vi "Update All.vi"(0 "reference in":refnum<class "AI.lvclass">, 5 "error in (no error)":errorcluster) -> (14 "reference out":refnum<class "AI.lvclass">, 19 "error out":errorcluster)   [LabVIEW 2017, in "AI.lvclass"]
uses:
  AI.lvclass
  <vilib>/DAQmx/read.llb/DAQmx Read (Analog 2D DBL NChan NSamp).vi
  <vilib>/DAQmx/miscellaneous.llb/DAQmx Fill In Error Info.vi
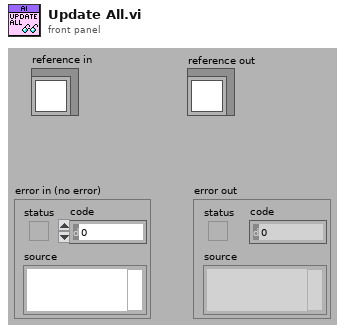
[diagram p1: front panel]
types:
  T1 = typedef "AI.lvclass/ObjectAttributes.ctl" = cluster{"AI Task":refnum<k21>, "AI On/Off Status":bool, "AI Sampling Rate (Samples/Seconds)":u32, "Number of AI Samples Per Channel":i32, "AI Voltage Range":u8, "AI Readings":dbl[][], "Number of AI Modules":i32, "Number of Total AI Channels":i32, "AI Module Names (NI-Max Name)":string[], "Number of Channels Per AI  Module":i32[], "AI VI Reference":refnum<vi>}
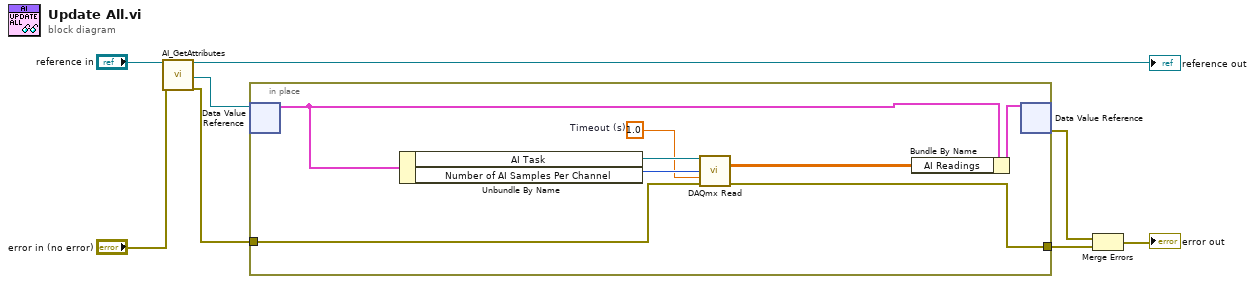
[diagram p0: block diagram]
diagram:
  n1 = call "AI_GetAttributes.vi"("reference in"="reference in", "error in (no error)"="error in (no error)") -> ("reference out"=→"reference out":refnum<class "AI.lvclass">, "DataRef"=w3:refnum<data-value>, "error out"=w1:errorcluster)  [unwired: 14 in, 1 out]
  n2 = in-place {
    in-place-border: [w10] -> w2
    in-place-border: w1 -> [w9]
    w13 = 1.0  # Timeout (s)
    n3 = in-place-dvr #1(w3) -> (w12:T1)  [unwired: 1 out]
    n4 = Unbundle By Name(w12) -> ("AI Task"=w15:refnum<k21>, "Number of AI Samples Per Channel"=w14:i32)
    n5 = call-poly <vilib>:"DAQmx Read.vi"("task/channels in"=w15, "number of samples per channel"=w14, "timeout"=w13, "error in"=w9) -> ("data"=w11:dbl[][], "error out"=w10:errorcluster)  [unwired: 9 in, 1 out]
    n6 = Bundle By Name(cluster=w12, "AI Readings"=w11) -> (w16:T1)
    n7 = in-place-dvr #1(w16) -> (w4:errorcluster)  [unwired: 1 out]
  }
  n8 = Merge Errors(w4, w2) -> (→"error out":errorcluster)
